vi "Tabor 5064 - Get Channel Status (SubVI).vi"(5 "error_in":errorcluster, 6 "GPIB Address":string="4", 7 "write_delay (ms)":u32=100, 9 "read_delay (ms)":u32=100) -> (14 "ch_status":bool[](array[boolean]), 15 "amps":dbl[](array[numeric]), 16 "offsets":dbl[](array[numeric]), 17 "freqs":dbl[](array[numeric]), 18 "phases":dbl[](array[numeric]), 19 "error_out":errorcluster)   [LabVIEW 2022 SP3]
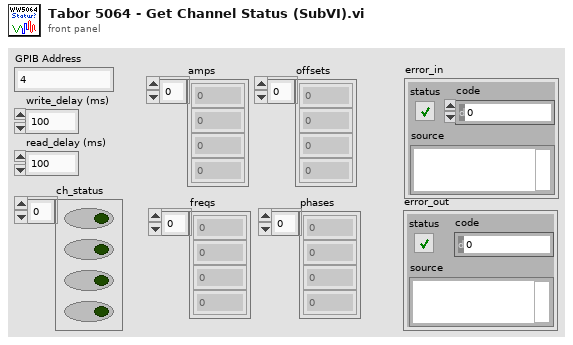
[diagram p1: front panel]
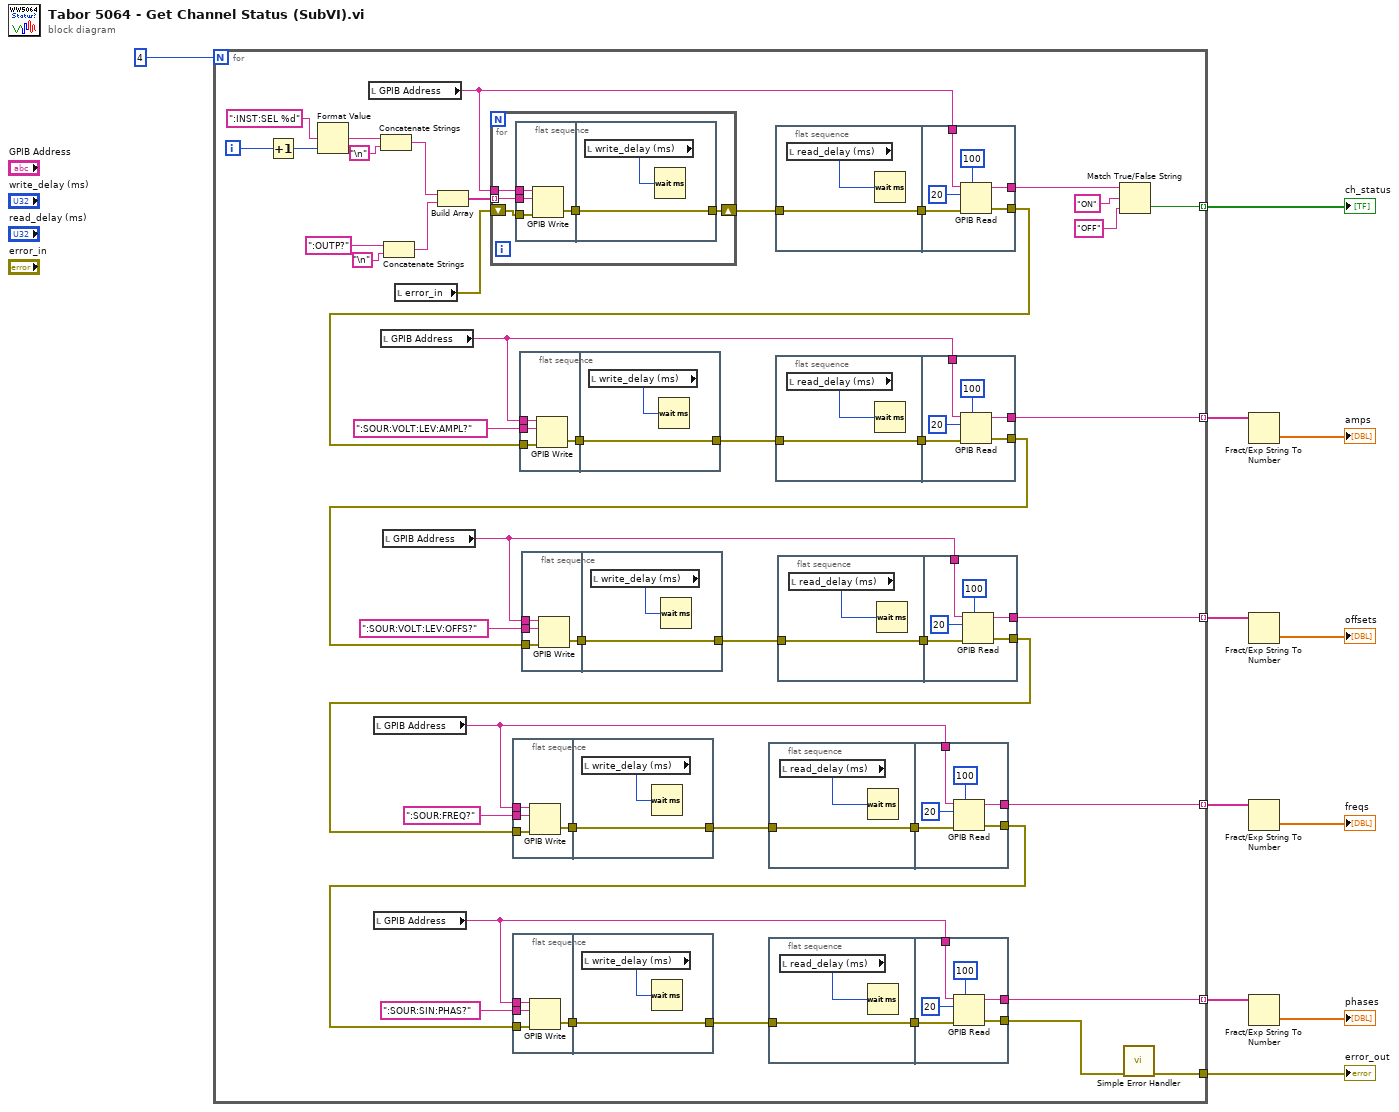
[diagram p0: block diagram]
diagram:
  n1 = for {
    N: 4 -> [_]
    tunnel: [w45] -> w11 mode=indexing
    tunnel: [w20] -> w8 mode=indexing
    tunnel: [w19] -> w5 mode=indexing
    tunnel: [w18] -> w4 mode=indexing
    tunnel: [w17] -> w2 mode=indexing
    tunnel: [w16] -> w9
    i -> [w51]
    n2 = Increment(x=w51) -> (x+1=w57:i32)
    n3 = Format Value(format string=":INST:SEL %d", value (0)=w57) -> (output string=w58:string)  [unwired: 1 in]
    n4 = local read "GPIB Address"() -> (w43:string)
    n5 = local read "GPIB Address"() -> (w26:string)
    n6 = local read "GPIB Address"() -> (w21:string)
    n7 = Concatenate Strings(w58, "\n") -> (w53:string)
    n8 = local read "GPIB Address"() -> (w36:string)
    n9 = local read "GPIB Address"() -> (w31:string)
    n10 = Concatenate Strings(":OUTP?" ("format string"), "\n") -> (w52:string)
    n11 = local read "error_in"() -> (w42:errorcluster)
    n12 = Build Array(w53, w52) -> (w50:string[])
    n13 = for {
      tunnel: w43 -> [w127]
      tunnel: w50 -> [w126] mode=indexing
      shift-right: [w125] -> w49
      shift-left: w42 -> [w124]
      n14 = flat-sequence {
        tunnel: w127 -> [w131]
        tunnel: w126 -> [w130]
        tunnel: w124 -> [w128]
        tunnel: [w129] -> w123
        tunnel: [w133] -> w125
        tunnel: w123 -> [w133]
        frame #0 {
          n15 = GPIB Write(0:w131, 1:w130, 3:w128) -> (6:w129:errorcluster)  [unwired: 2 in, 1 out]
        }
        frame #1 {
          n16 = local read "write_delay (ms)"() -> (w132:u32)
          n17 = Wait (ms)(milliseconds to wait=w132) -> ()  [unwired: 1 out]
        }
      }
    }
    n18 = flat-sequence {
      tunnel: w26 -> [w84]
      tunnel: w13 -> [w82]
      tunnel: [w83] -> w30
      tunnel: ":SOUR:FREQ?" ("format string") -> [w81]
      tunnel: [w86] -> w27
      tunnel: w30 -> [w86]
      frame #0 {
        n19 = GPIB Write(0:w84, 1:w81, 3:w82) -> (6:w83:errorcluster)  [unwired: 2 in, 1 out]
      }
      frame #1 {
        n20 = local read "write_delay (ms)"() -> (w85:u32)
        n21 = Wait (ms)(milliseconds to wait=w85) -> ()  [unwired: 1 out]
      }
    }
    n22 = flat-sequence {
      tunnel: w21 -> [w70]
      tunnel: w12 -> [w68]
      tunnel: [w69] -> w25
      tunnel: ":SOUR:SIN:PHAS?" ("format string") -> [w67]
      tunnel: [w72] -> w22
      tunnel: w25 -> [w72]
      frame #0 {
        n23 = GPIB Write(0:w70, 1:w67, 3:w68) -> (6:w69:errorcluster)  [unwired: 2 in, 1 out]
      }
      frame #1 {
        n24 = local read "write_delay (ms)"() -> (w71:u32)
        n25 = Wait (ms)(milliseconds to wait=w71) -> ()  [unwired: 1 out]
      }
    }
    n26 = flat-sequence {
      tunnel: w36 -> [w112]
      tunnel: w15 -> [w110]
      tunnel: [w111] -> w40
      tunnel: ":SOUR:VOLT:LEV:AMPL?" ("format string") -> [w109]
      tunnel: [w114] -> w37
      tunnel: w40 -> [w114]
      frame #0 {
        n27 = GPIB Write(0:w112, 1:w109, 3:w110) -> (6:w111:errorcluster)  [unwired: 2 in, 1 out]
      }
      frame #1 {
        n28 = local read "write_delay (ms)"() -> (w113:u32)
        n29 = Wait (ms)(milliseconds to wait=w113) -> ()  [unwired: 1 out]
      }
    }
    n30 = flat-sequence {
      tunnel: w31 -> [w98]
      tunnel: w14 -> [w96]
      tunnel: [w97] -> w35
      tunnel: ":SOUR:VOLT:LEV:OFFS?" ("format string") -> [w95]
      tunnel: [w100] -> w32
      tunnel: w35 -> [w100]
      frame #0 {
        n31 = GPIB Write(0:w98, 1:w95, 3:w96) -> (6:w97:errorcluster)  [unwired: 2 in, 1 out]
      }
      frame #1 {
        n32 = local read "write_delay (ms)"() -> (w99:u32)
        n33 = Wait (ms)(milliseconds to wait=w99) -> ()  [unwired: 1 out]
      }
    }
    n34 = flat-sequence {
      tunnel: w27 -> [w74]
      tunnel: [w74] -> w29
      tunnel: w26 -> [w79]
      tunnel: [w77] -> w12
      tunnel: [w76] -> w18
      tunnel: w29 -> [w80]
      frame #0 {
        n35 = local read "read_delay (ms)"() -> (w73:u32)
        n36 = Wait (ms)(milliseconds to wait=w73) -> ()  [unwired: 1 out]
      }
      frame #1 {
        n37 = GPIB Read(0:w79, 1:20 ("byte count"), 3:w80, 4:100 ("timeout ms (488.2 global)")) -> (5:w76:string, 7:w77:errorcluster)  [unwired: 1 in, 1 out]
      }
    }
    n38 = flat-sequence {
      tunnel: w22 -> [w60]
      tunnel: [w60] -> w24
      tunnel: w21 -> [w65]
      tunnel: [w63] -> w16
      tunnel: [w62] -> w17
      tunnel: w24 -> [w66]
      frame #0 {
        n39 = local read "read_delay (ms)"() -> (w59:u32)
        n40 = Wait (ms)(milliseconds to wait=w59) -> ()  [unwired: 1 out]
      }
      frame #1 {
        n41 = GPIB Read(0:w65, 1:20 ("byte count"), 3:w66, 4:100 ("timeout ms (488.2 global)")) -> (5:w62:string, 7:w63:errorcluster)  [unwired: 1 in, 1 out]
      }
    }
    n42 = flat-sequence {
      tunnel: w49 -> [w116]
      tunnel: [w116] -> w44
      tunnel: w43 -> [w121]
      tunnel: [w119] -> w15
      tunnel: [w118] -> w46
      tunnel: w44 -> [w122]
      frame #0 {
        n43 = local read "read_delay (ms)"() -> (w115:u32)
        n44 = Wait (ms)(milliseconds to wait=w115) -> ()  [unwired: 1 out]
      }
      frame #1 {
        n45 = GPIB Read(0:w121, 1:20 ("byte count"), 3:w122, 4:100 ("timeout ms (488.2 global)")) -> (5:w118:string, 7:w119:errorcluster)  [unwired: 1 in, 1 out]
      }
    }
    n46 = flat-sequence {
      tunnel: w37 -> [w102]
      tunnel: [w102] -> w38
      tunnel: w36 -> [w107]
      tunnel: [w105] -> w14
      tunnel: [w104] -> w20
      tunnel: w38 -> [w108]
      frame #0 {
        n47 = local read "read_delay (ms)"() -> (w101:u32)
        n48 = Wait (ms)(milliseconds to wait=w101) -> ()  [unwired: 1 out]
      }
      frame #1 {
        n49 = GPIB Read(0:w107, 1:20 ("byte count"), 3:w108, 4:100 ("timeout ms (488.2 global)")) -> (5:w104:string, 7:w105:errorcluster)  [unwired: 1 in, 1 out]
      }
    }
    n50 = flat-sequence {
      tunnel: w32 -> [w88]
      tunnel: [w88] -> w34
      tunnel: w31 -> [w93]
      tunnel: [w91] -> w13
      tunnel: [w90] -> w19
      tunnel: w34 -> [w94]
      frame #0 {
        n51 = local read "read_delay (ms)"() -> (w87:u32)
        n52 = Wait (ms)(milliseconds to wait=w87) -> ()  [unwired: 1 out]
      }
      frame #1 {
        n53 = GPIB Read(0:w93, 1:20 ("byte count"), 3:w94, 4:100 ("timeout ms (488.2 global)")) -> (5:w90:string, 7:w91:errorcluster)  [unwired: 1 in, 1 out]
      }
    }
    n54 = Match True/False String(2:"OFF" ("false string"), 3:"ON" ("true string"), 4:w46) -> (0:w45:bool)  [unwired: 1 out]
    n55 = call <vilib>:"Simple Error Handler.vi"("error in (no error)"=w16) -> ()  [unwired: 4 in, 5 out]
  }
  "ch_status" <- w11
  "error_out" <- w9
  n56 = Fract/Exp String To Number(string=w8) -> (number=→"amps":dbl[])  [unwired: 3 in, 1 out]
  n57 = Fract/Exp String To Number(string=w5) -> (number=→"offsets":dbl[])  [unwired: 3 in, 1 out]
  n58 = Fract/Exp String To Number(string=w4) -> (number=→"freqs":dbl[])  [unwired: 3 in, 1 out]
  n59 = Fract/Exp String To Number(string=w2) -> (number=→"phases":dbl[])  [unwired: 3 in, 1 out]
